vi "Ondas.vi"() -> ()   [LabVIEW 2020]
uses:
  <vilib>/measure/NI_MABase.lvlib
panel:
  in  "Knob 6":dbl(knob) scale=0.0..10.0
  in  "Knob 5":dbl(knob) scale=0.0..100.0
  in  "Knob 4":dbl(knob) scale=0.0..100.0
  in  "Knob 3":dbl(knob) scale=0.0..100.0
  in  "Knob 2":dbl(knob) scale=0.0..100.0
  in  "Knob":dbl(knob) scale=0.0..100.0
  out "XY Graph 2":cluster{"Y":dbl[], "Y":dbl[]}[](graph)
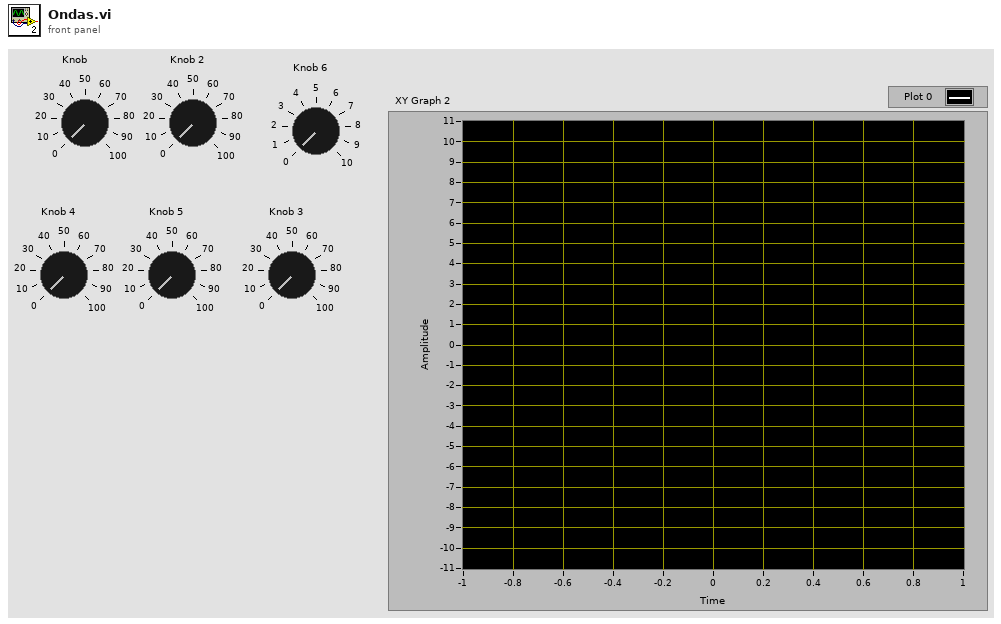
[diagram p1: front panel]
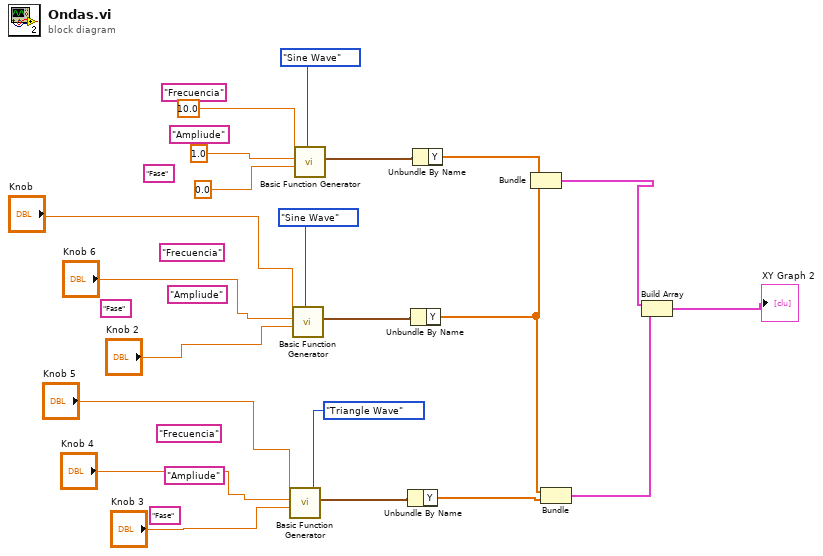
[diagram p0: block diagram]
diagram:
  (unwired) "Fase"
  (unwired) "Ampliude"
  (unwired) "Frecuencia"
  (unwired) "Fase"
  (unwired) "Ampliude"
  (unwired) "Frecuencia"
  (unwired) "Fase"
  (unwired) "Ampliude"
  (unwired) "Frecuencia"
  n1 = call <vilib>:"Basic Function Generator.vi"("signal type"=enum16{"Sine Wave", "Triangle Wave"}."Triangle Wave", "phase"="Knob 3", "amplitude"="Knob 4", "frequency"="Knob 5") -> ("signal out"=w14:waveform(dbl))  [unwired: 5 in, 2 out]
  n2 = call <vilib>:"Basic Function Generator.vi"("signal type"=enum16{"Sine Wave"}."Sine Wave", "phase"="Knob 2", "amplitude"="Knob 6", "frequency"="Knob") -> ("signal out"=w15:waveform(dbl))  [unwired: 5 in, 2 out]
  n3 = call <vilib>:"Basic Function Generator.vi"("signal type"=enum16{"Sine Wave"}."Sine Wave", "phase"=0.0, "amplitude"=1.0, "frequency"=10.0) -> ("signal out"=w18:waveform(dbl))  [unwired: 5 in, 2 out]
  n4 = Unbundle By Name(w14) -> ("Y"=w12:dbl[])
  n5 = Unbundle By Name(w15) -> ("Y"=w11:dbl[])
  n6 = Unbundle By Name(w18) -> ("Y"=w17:dbl[])
  n7 = Bundle("Y"=w17, "Y"=w11) -> (w10:cluster{"Y":dbl[], "Y":dbl[]})  [unwired: 1 in]
  n8 = Bundle("Y"=w11, "Y"=w12) -> (w9:cluster{"Y":dbl[], "Y":dbl[]})  [unwired: 1 in]
  n9 = Build Array(w10, w9) -> (→"XY Graph 2":cluster{"Y":dbl[], "Y":dbl[]}[])
